vi "JKISM++ Destroy Status Change Event.vi"(8 "Error in":errorcluster caption="Error in (no error)", 11 "Status Change Event":refnum<user-event>) -> (0 "Error out":errorcluster)   [LabVIEW 2014, in "JKI State Machine++.lvlib"]
doc: "Release JKISM++ Global Log Event Reference.\n\n<b>Inputs:</b>\n - <b>JKISM Global Log Event</b>:\n - <b>Error in</b>: Error cluster\n\n<b>Outputs:</b>\n - <b>Error out</b>: Error cluster"
uses:
  JKI State Machine++.lvlib
  _Support/Typedef/_JKISM Status Change Event Data.ctl
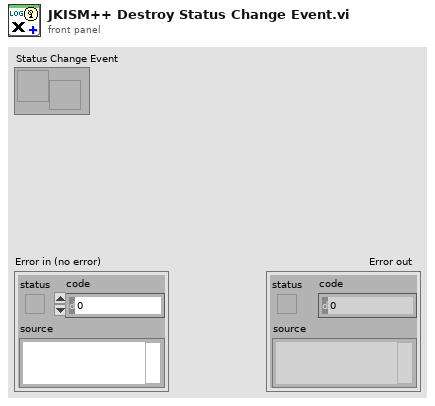
[diagram p1: front panel]
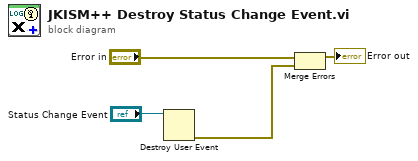
[diagram p0: block diagram]
diagram:
  n1 = Destroy User Event(user event="Status Change Event") -> (error out=w4:errorcluster)  [unwired: 1 in]
  n2 = Merge Errors("Error in", w4) -> (→"Error out":errorcluster)
